vi "LVClass_Camera get image.vi"(0 "Camera in":refnum<class "Camera.lvclass">, 5 "Image":refnum<class "Image.lvclass">, 7 "Image RAW":refnum<class "Image.lvclass">, 9 "remove_background":bool=TRUE, 11 "error in (no error)":errorcluster) -> (4 "Camera out":refnum<class "Camera.lvclass">, 6 "Image (dup)":refnum<class "Image.lvclass">, 8 "Image (dup) RAW":refnum<class "Image.lvclass">, 15 "error out":errorcluster)   [LabVIEW 2020, in "Camera.lvclass"]
doc: "Retrieve last captured image. see Imop_Camera_AsyncImageReady.\n\n<B>CameraIn</B> : Camera object.\n<B>CameraOut</B> : Camera object.\n<B>Image</B> : Captured image with (optionnally) background removed.\n<B>remove_background</B> : Boolean which indicates if background should be substracted.\n<B>RawImage</B> : Captured image without any post-processing applied."
uses:
  Camera.lvclass
  Image.lvclass
  Camera.lvclass/Camera.ctl
  CameraAcquisitionState.ctl
  LVClass_Image read Image Compat ptr.vi
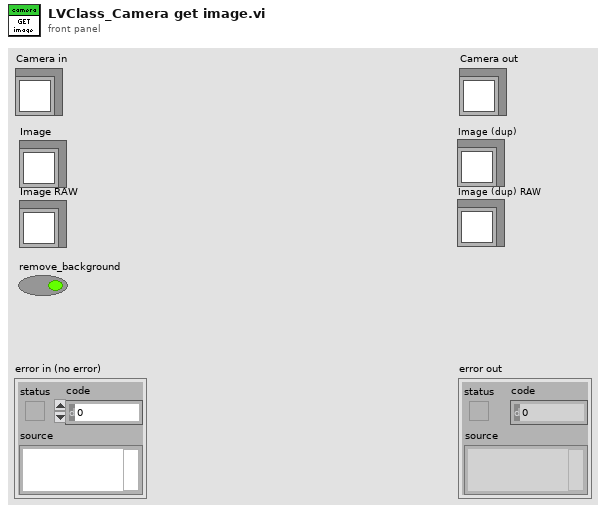
[diagram p1: front panel]
types:
  T1 = typedef "CameraAcquisitionState.ctl" = enum16{"Stop", "Live"}
  T2 = typedef "ClassID.ctl" = i64
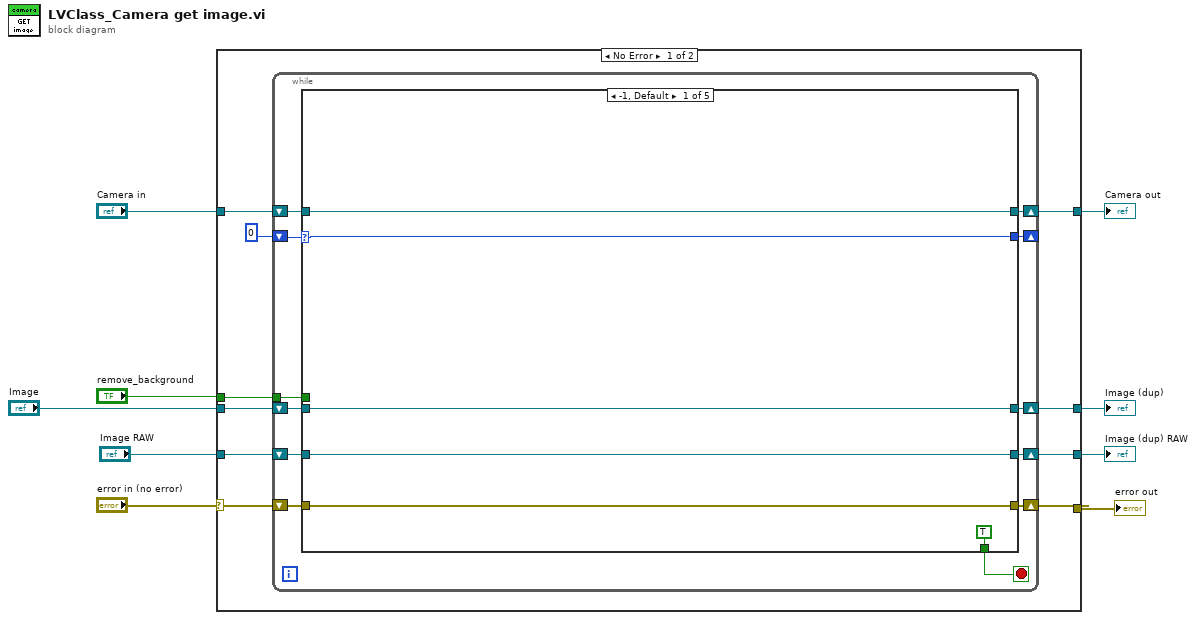
[diagram p0: block diagram]
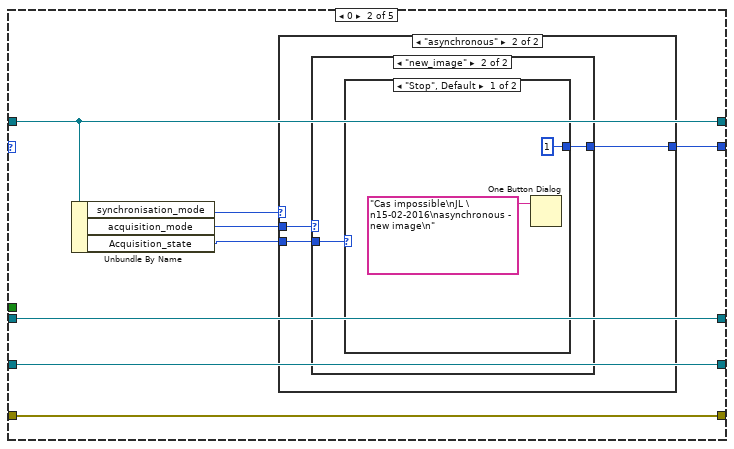
[diagram p2: hidden frame]
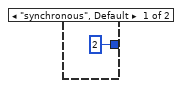
[diagram p3: hidden frame]
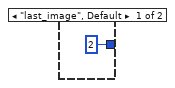
[diagram p4: hidden frame]
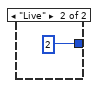
[diagram p5: hidden frame]
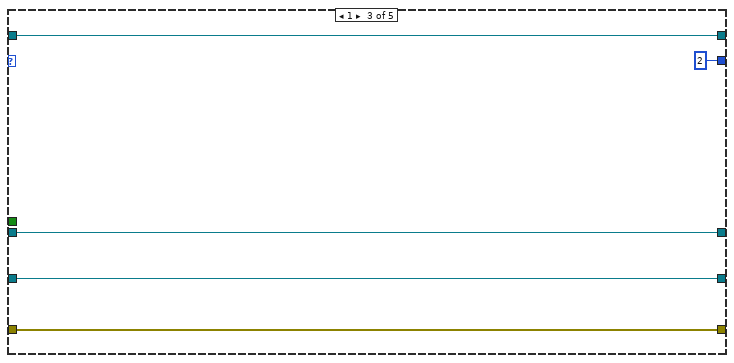
[diagram p6: hidden frame]
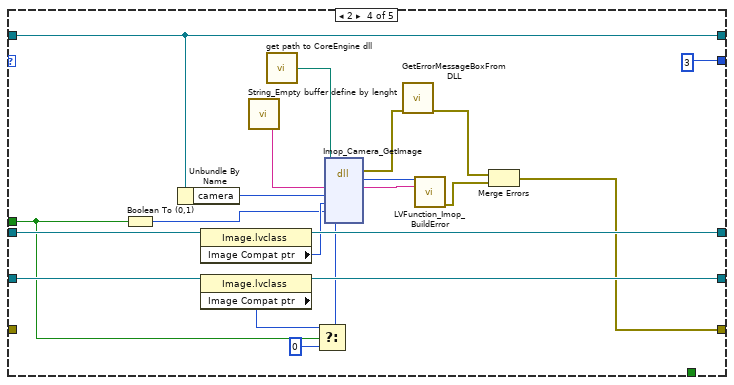
[diagram p7: hidden frame]
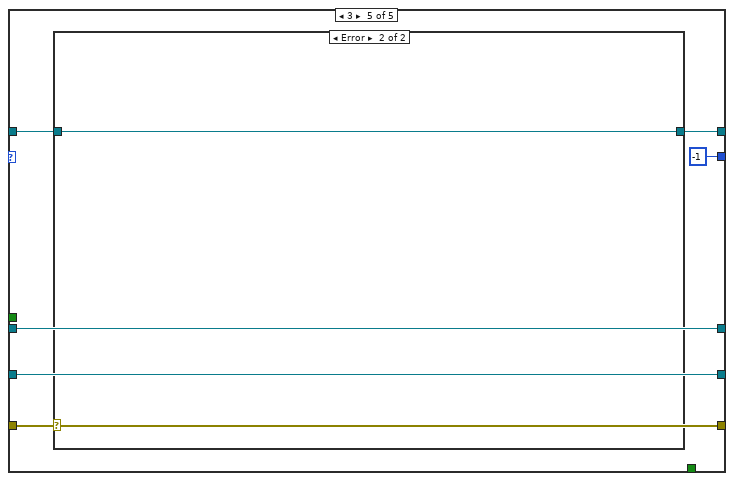
[diagram p8: hidden frame]
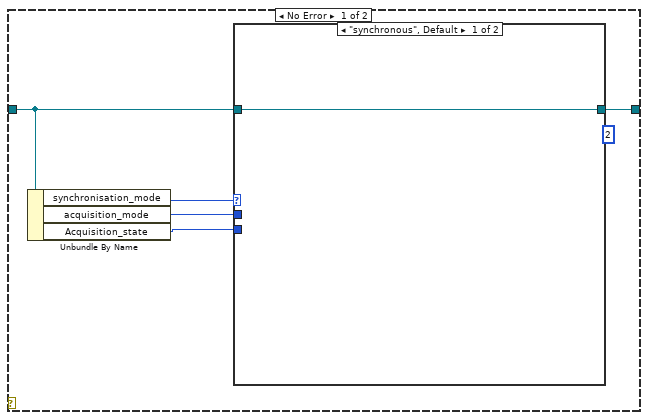
[diagram p9: hidden frame]
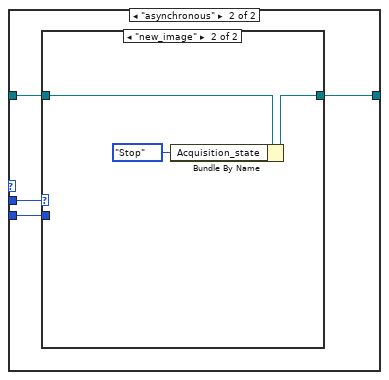
[diagram p10: hidden frame]
diagram:
  n1 = case shown="No Error" "error in (no error)" {
    selector: "error in (no error)" -> [w12 w106]
    tunnel: [w14 w106] -> w8
    tunnel: [w10 w105] -> w6
    tunnel: "Camera in" -> [w11 w105]
    tunnel: [w18 w104] -> w5
    tunnel: "Image" -> [w19 w104]
    tunnel: "Image RAW" -> [w17 w103]
    tunnel: [w16 w103] -> w2
    tunnel: "remove_background" -> [w15 _]
    frame No Error {
      n2 = while {
        tunnel: w15 -> [w27]
        shift-right: [w23] -> w10
        shift-left: w11 -> [w25]
        shift-right: [w30] -> w18
        shift-left: w19 -> [w31]
        shift-right: [w28] -> w16
        shift-left: w17 -> [w29]
        shift-right: [w26] -> w14
        shift-left: w12 -> [w22]
        shift-right: [w21] -> _
        shift-left: 0 -> [w24]
        stop <- w20 stop-if-true
        n3 = case shown="-1, Default" w24 {
          selector: w24 -> [w33 _ _ _ _]
          tunnel: w31 -> [w35 w39 w60 w81 w87]
          tunnel: [w35 w39 w60 w80 w87] -> w30
          tunnel: w29 -> [w34 w38 w59 w79 w86]
          tunnel: [w34 w38 w59 w78 w86] -> w28
          tunnel: w27 -> [_ _ _ w64 _]
          tunnel: [w37 w45 w56 w77 w82] -> w26
          tunnel: w25 -> [w36 w44 w57 w76 w84]
          tunnel: [w36 w44 w57 w76 w85] -> w23
          tunnel: w22 -> [w37 w45 w56 _ w82]
          tunnel: [w33 w40 2 3 -1] -> w21
          tunnel: [TRUE _ _ _ _] -> w20
          frame -1, Default {
          }
          frame 0 {
            n4 = Unbundle By Name(w44) -> ("synchronisation_mode"=w43:enum16{"synchronous", "asynchronous"}, "acquisition_mode"=w42:enum16{"last_image", "new_image"}, "Acquisition_state"=w41:T1)
            n5 = case shown="\"asynchronous\"" w43 {
              tunnel: w42 -> [_ w49]
              tunnel: w41 -> [_ w48]
              tunnel: [2 w47] -> w40
              frame "synchronous", Default {
              }
              frame "asynchronous" {
                n6 = case shown="\"new_image\"" w49 {
                  tunnel: w48 -> [_ w52]
                  tunnel: [2 w51] -> w47
                  frame "last_image", Default {
                  }
                  frame "new_image" {
                    n7 = case shown="\"Stop\", Default" w52 {
                      tunnel: [1 2] -> w51
                      frame "Stop", Default {
                        n8 = One Button Dialog(message="Cas impossible\nJL \n15-02-2016\nasynchronous - new image\n") -> ()  [unwired: 1 in, 1 out]
                      }
                      frame "Live" {
                      }
                    }
                  }
                }
              }
            }
          }
          frame 1 {
          }
          frame 2 {
            n9 = Boolean To (0,1)(Boolean=w64) -> (0, 1=w67:i16)
            n10 = Unbundle By Name(w76) -> ("camera"=w71:T2)
            n11 = property class="Image.lvclass"(reference=w81) -> (reference out=w80:refnum<class "Image.lvclass">, "Image Compat ptr"=w69:T2)  [unwired: 1 in, 1 out]
            n12 = property class="Image.lvclass"(reference=w79) -> (reference out=w78:refnum<class "Image.lvclass">, "Image Compat ptr"=w62:T2)  [unwired: 1 in, 1 out]
            n13 = call "String_Empty buffer define by lenght.vi"() -> ("Empty buffer"=w74:string)  [unwired: 1 in]
            n14 = call "get path to CoreEngine dll.vi"() -> ("path to wavekit library"=w70:path)  [unwired: 14 in, 1 out]
            n15 = Select(t=w62, s=w64, f=0) -> (s? t:f=w61:T2)
            n16 = dll-call lib="D:/soft/HASO_v3/SVN_trunk/ImOpCoreEngine4_LV2011/DLLs/c_interface_vc100.dll" fn="Imop_Camera_GetImage"(path in=w70, "message"=w74, "camera"=w71, "HASO_image"=w69, "remove background"=w67, "RAW HASO_image"=w61) -> (error out=w68:errorcluster, "return type"=w73:i32, "message"=w72:string)  [unwired: 6 in, 1 out]
            n17 = call "GetErrorMessageBoxFromDLL.vi"("error IN"=w68) -> ("error OUT"=w66:errorcluster)  [unwired: 10 in]
            n18 = call "LVFunction_Imop_BuildError.vi"("code"=w73, "String to Prepend to source (\"\")"=w72) -> ("error out"=w65:errorcluster)  [unwired: 13 in]
            n19 = Merge Errors(w66, w65) -> (w77:errorcluster)
          }
          frame 3 {
            n20 = case shown="Error" w82 {
              tunnel: [w89 w102] -> w85
              tunnel: w84 -> [w88 w102]
              frame No Error {
                n21 = Unbundle By Name(w88) -> ("synchronisation_mode"=w92:enum16{"synchronous", "asynchronous"}, "acquisition_mode"=w91:enum16{"last_image", "new_image"}, "Acquisition_state"=w90:T1)
                n22 = case shown="\"synchronous\", Default" w92 {
                  tunnel: w91 -> [_ w97]
                  tunnel: w90 -> [_ w96]
                  tunnel: [w93 w95] -> w89
                  tunnel: w88 -> [w93 w94]
                  frame "synchronous", Default {
                    (unwired) 2
                  }
                  frame "asynchronous" {
                    n23 = case shown="\"new_image\"" w97 {
                      tunnel: w96 -> [_ _]
                      tunnel: [w98 w99] -> w95
                      tunnel: w94 -> [w98 w100]
                      frame "last_image", Default {
                      }
                      frame "new_image" {
                        n24 = Bundle By Name(cluster=w100, "Acquisition_state"=CameraAcquisitionState."Stop") -> (w99:refnum<class "Camera.lvclass">)
                      }
                    }
                  }
                }
              }
              frame Error {
              }
            }
          }
        }
      }
    }
    frame Error {
    }
  }
  "error out" <- w8
  "Camera out" <- w6
  "Image (dup)" <- w5
  "Image (dup) RAW" <- w2
